vi "Global display 1.vi"() -> ()   [LabVIEW 2013]
panel:
  in  "TEST 5-2":T1(radio)
  in  "TEST 5-1":T1(radio)
  in  "TEST 4-2":T1(radio)
  in  "TEST 4-1":T1(radio)
  in  "TEST 3-2":T1(radio)
  in  "TEST 3-1":T1(radio)
  in  "TEST 2-2":T1(radio)
  in  "TEST 2-1":T1(radio)
  in  "TEST 1-2":T1(radio)
  in  "TEST 1-1":T1(radio)
  out "5-2 R/S":bool
  out "5-2 O/F":bool
  out "5-1 R/S":bool
  out "5-1 O/F":bool
  out "4-2 R/S":bool
  out "4-2 O/F":bool
  out "4-1 R/S":bool
  out "4-1 O/F":bool
  out "3-2 R/S":bool
  out "3-2 O/F":bool
  out "3-1 R/S":bool
  out "3-1 O/F":bool
  out "2-2 R/S":bool
  out "2-2 O/F":bool
  out "2-1 R/S":bool
  out "2-1 O/F":bool
  out "1-2 R/S":bool
  out "1-2 O/F":bool
  out "1-1 R/S":bool
  out "1-1 O/F":bool
  out "SIG LAB05-2":T2 {"PF" format="%.2f"; "AMPS" format="%.1f"}
  out "SIG LAB05-1":T2 {"PF" format="%.2f"; "AMPS" format="%.1f"}
  out "SIG LAB04-2":T2 {"PF" format="%.2f"; "AMPS" format="%.1f"}
  out "SIG LAB04-1":T2 {"PF" format="%.2f"; "AMPS" format="%.1f"}
  out "SIG LAB03-2":T2 {"PF" format="%.2f"; "AMPS" format="%.1f"}
  out "SIG LAB03-1":T2 {"PF" format="%.2f"; "AMPS" format="%.1f"}
  out "SIG LAB02-2":T2 {"PF" format="%.2f"; "AMPS" format="%.1f"}
  out "SIG LAB02-1":T2 {"PF" format="%.2f"; "AMPS" format="%.1f"}
  out "SIG LAB01-2":T2 {"PF" format="%.2f"; "AMPS" format="%.1f"}
  out "SIG LAB01-1":T2 {"PF" format="%.2f"; "AMPS" format="%.1f"}
  out "stop disp":bool
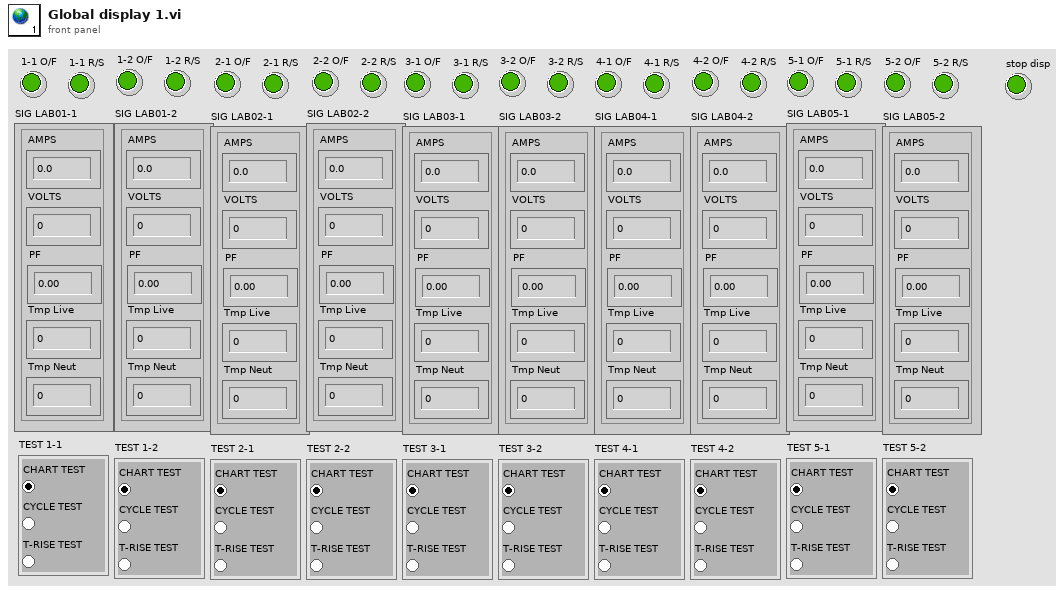
[diagram p1: front panel]
types:
  T1 = enum32{"CHART TEST", "CYCLE TEST", "T-RISE TEST"}
  T2 = cluster{"AMPS":dbl, "VOLTS":dbl, "PF":dbl, "Tmp Live":dbl, "Tmp Neut":dbl}
diagram:
